vi "Create.vi"(8 "error in (no error)":errorcluster) -> (0 "error out":errorcluster, 3 "Parallell Test Runner out":refnum<class "Parallel Test Runner.lvclass">)   [LabVIEW 2020, in "Parallel Test Runner.lvclass"]
uses:
  Parallel Test Runner.lvclass
  Parallel Test Runner.lvclass/Parallel Test Runner.ctl
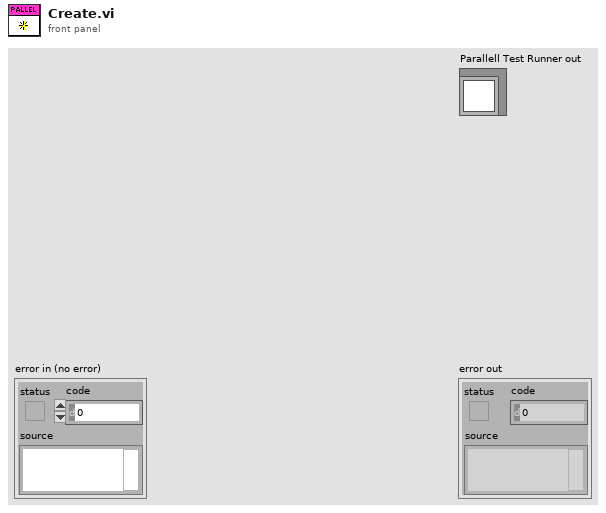
[diagram p1: front panel]
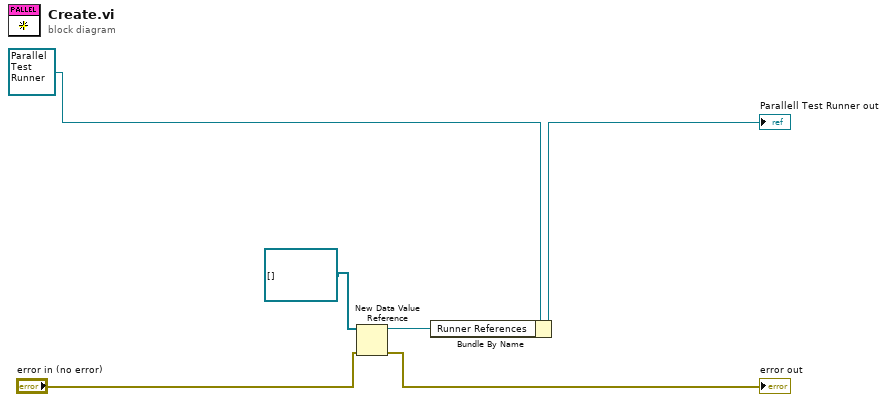
[diagram p0: block diagram]
diagram:
  n1 = New Data Value Reference(data value=refnum<vi>[] [], error in="error in (no error)") -> (data value reference=w3:refnum<data-value>, error out=→"error out":errorcluster)
  n2 = Bundle By Name(cluster=refnum<class "Parallel Test Runner.lvclass"> refnum ("Parallell Test Runner in"), "Runner References"=w3) -> (→"Parallell Test Runner out":refnum<class "Parallel Test Runner.lvclass">)
